vi "Minimal AR Example - Render 3D.vi"(6 "Camera Parameters":T5, 8 "error in (no error)":errorcluster, 10 "Pose":T1, 11 "ARGB Image In":T4) -> (0 "error out":errorcluster, 3 "ARGB Image Out":T4)   [LabVIEW 2020, in "examples.lvlib"]
uses:
  examples.lvlib
  common/Camera Parameters.ctl
  common/Camera Matrix.ctl
  common/Camera Distortion Coefficients.ctl
  image/ARGB Image.ctl
  ar/Pose.ctl
  ar/rvec.ctl
  ar/tvec.ctl
  image/Copy Pixmap to Image (ARGB Flatten Mask).vi
  image/Match-Value Image (Colour).vi
  image/Invert In-Place (Greyscale Bitwise).vi
  image/Copy Image (ARGB with Greyscale Mask).vi
  image/Size (ARGB).vi
  image/New Image (ARGB Preallocated).vi
  image/New Image (Greyscale Preallocated).vi
  ar/Rodrigues.vi
  ar/Rodrigues (RVec To RMat).vi
  ar/Transform Components to Transformation Matrix.vi
  <vilib>/Analysis/baseanly.llb/A x B.vi
  <vilib>/Analysis/baseanly.llb/Real A x B.vi
  image/ARGB Colour to U32 Pixel Value.vi
  image/Copy Pixmap to Image (ARGB Flatten Mask).vi/7d03ccf7-b889-4e8d-9f2a-57831e73dbde.vi
  image/Match-Value Image (Colour).vi/5701baee-35e2-4306-9a77-a9fdbb5b3a7f.vi
  image/Invert In-Place (Greyscale Bitwise).vi/821d400d-177f-4d99-a785-a8086a4d8ddd.vi
  image/Copy Image (ARGB with Greyscale Mask).vi/327a14ae-2acc-4952-87c0-fab6c3cd3da3.vi
  image/Size (ARGB).vi/69a1505b-b287-44ed-9ef9-f10ed7b260f4.vi
  image/New Image (ARGB Preallocated).vi/3321fa97-f432-4e1e-8db9-a0df79aed21b.vi
  image/New Image (Greyscale Preallocated).vi/6598b9e0-8a08-46f5-91fd-ca1b87217137.vi
  image/FixPixmap.vi
  image/Default8bitColourMap.vi
  <vilib>/Analysis/Matrix/Numeric/Conversions/Array To Matrix.vi
  <vilib>/Analysis/Matrix/Numeric/Conversions/Array To Matrix - RA2.vi
  <vilib>/Utility/error.llb/Error Cluster From Error Code.vi
  <vilib>/picture/3D Picture Control/Object/Create Object (name).vi
  <vilib>/picture/3D Picture Control/Object/Add Object (no reference).vi
  image/image.lvlib
  <vilib>/picture/3D Picture Control/NI_3D Picture Control.lvlib
  ar/ar.lvlib
  common/common.lvlib
panel:
  out "3D Canvas":refnum<vi>(3d-picture)
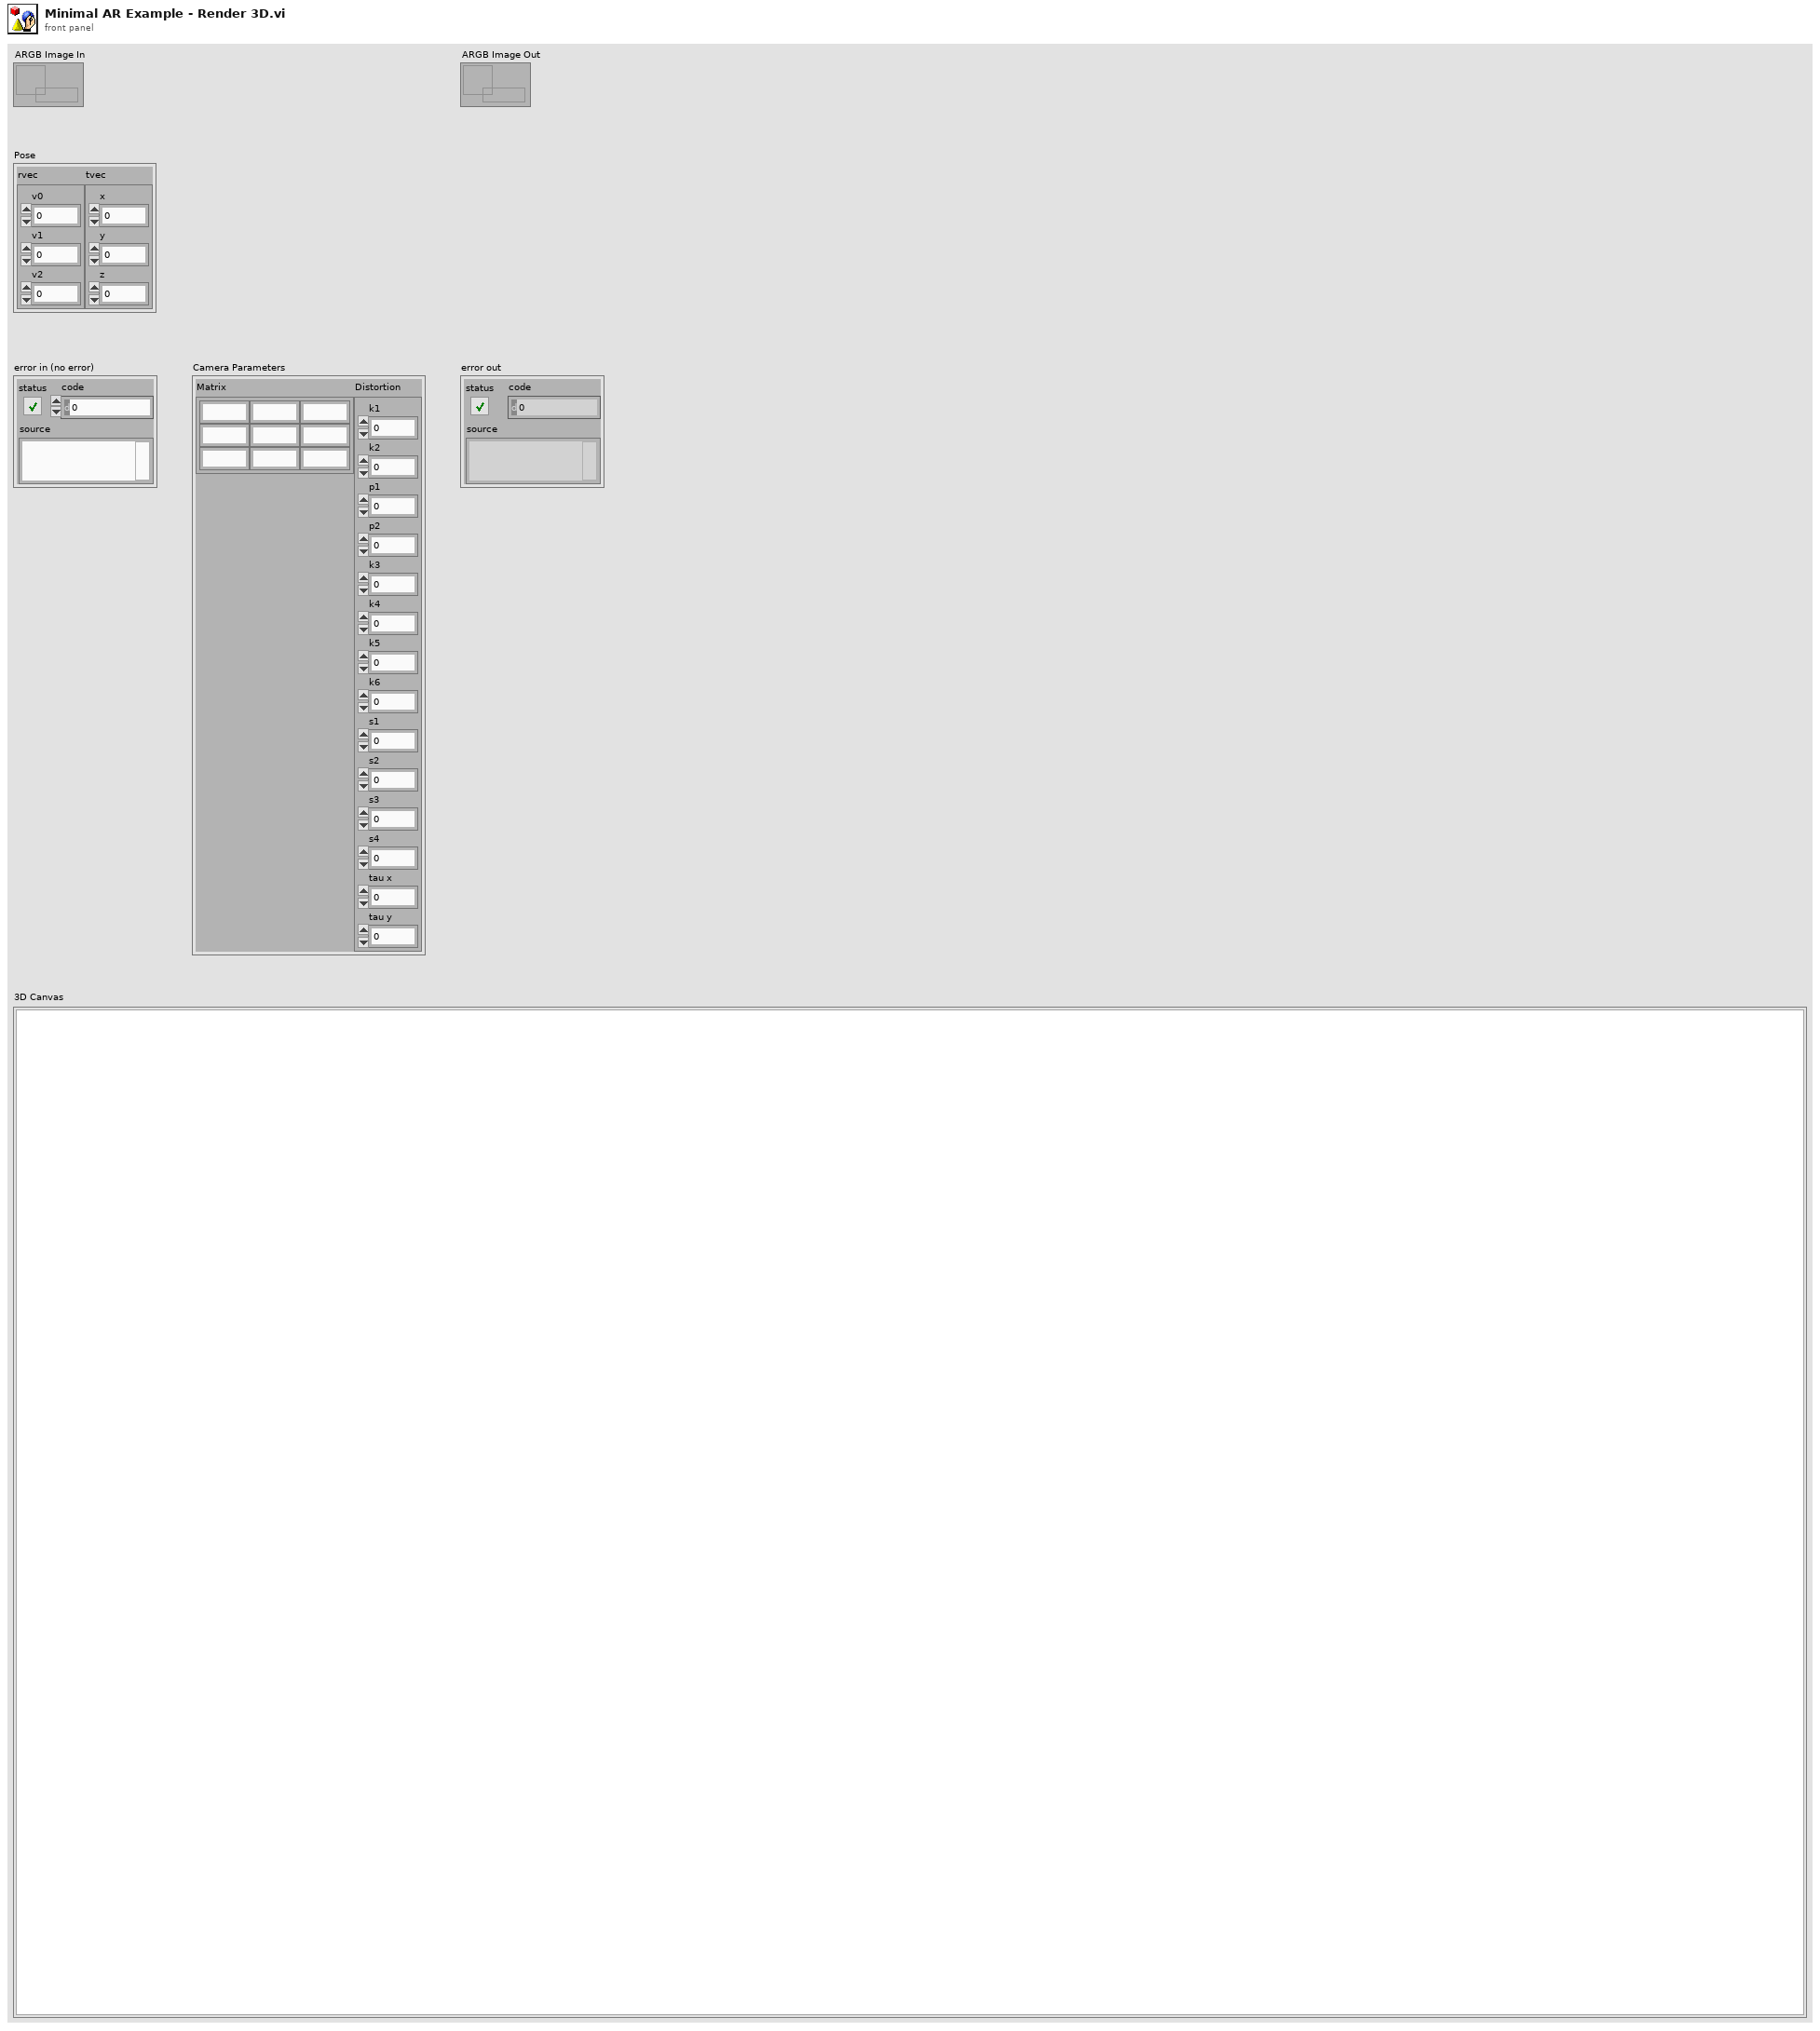
[diagram p1: front panel]
types:
  T1 = typedef "ar.lvlib/Pose.ctl" = cluster{"rvec":T2, "tvec":T3}
  T2 = typedef "ar.lvlib/rvec.ctl" = cluster{"v0":dbl, "v1":dbl, "v2":dbl}
  T3 = typedef "ar.lvlib/tvec.ctl" = cluster{"x":dbl, "y":dbl, "z":dbl}
  T4 = typedef "image.lvlib/ARGB Image.ctl" = refnum<data-value>
  T5 = typedef "common.lvlib/Camera Parameters.ctl" = cluster{"Matrix":T6, "Distortion":T7}
  T6 = typedef "common.lvlib/Camera Matrix.ctl" = cluster{"m 0,0":dbl, "m 0,1":dbl, "m 0,2":dbl, "m 1,0":dbl, "m 1,1":dbl, "m 1,2":dbl, "m 2,0":dbl, "m 2,1":dbl, "m 2,2":dbl}
  T7 = typedef "common.lvlib/Camera Distortion Coefficients.ctl" = cluster{"k1":dbl, "k2":dbl, "p1":dbl, "p2":dbl, "k3":dbl, "k4":dbl, "k5":dbl, "k6":dbl, "s1":dbl, "s2":dbl, "s3":dbl, "s4":dbl, "tau x":dbl, "tau y":dbl}
  T8 = typedef "NI_Matrix.lvlib/RealMatrix.ctl" = dbl[][]
  T9 = typedef "imagedata.ctl" = cluster{"image type":i32, "image depth":i32, "image":u8[], "mask":u8[], "colors":u32[], "Rectangle":cluster{"left":i16, "top":i16, "right":i16, "bottom":i16}}
  T10 = typedef "image.lvlib/Greyscale Image.ctl" = refnum<data-value>
  T11 = typedef "common.lvlib/Image Size (Integer).ctl" = cluster{"Width":u16, "Height":u16}
  T12 = typedef "LVBoundsTypeDef.ctl" = cluster{"Width":u32, "Height":u32}
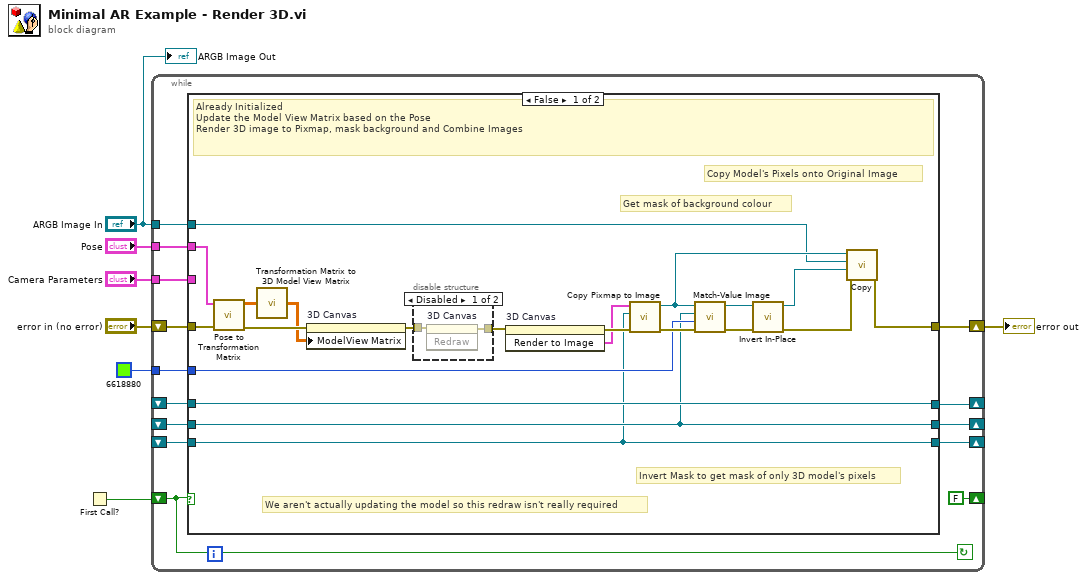
[diagram p0: block diagram]
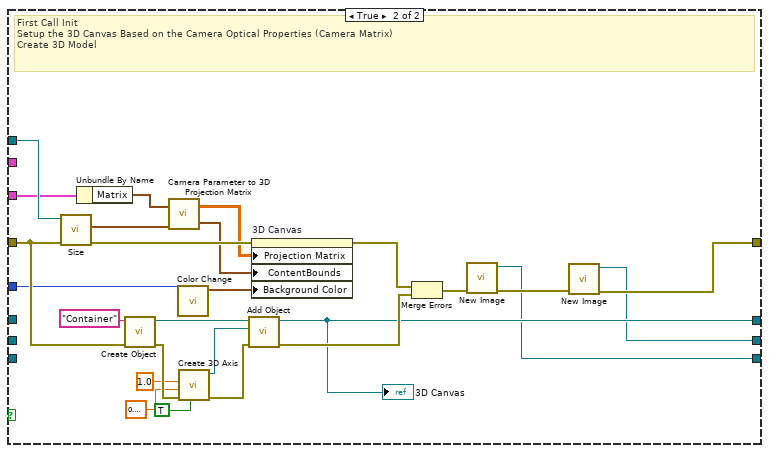
[diagram p3: hidden frame]
diagram:
  n1 = First Call?() -> (First Call?: T/F=w7:bool)
  n2 = while {
    shift-right: [FALSE ("First Call?: T/F")] -> _
    shift-left: w7 -> [w21]
    tunnel: "ARGB Image In" -> [w19]
    tunnel: "Camera Parameters" -> [w18]
    shift-right: [w14] -> w2
    shift-left: "error in (no error)" -> [w17]
    shift-right: [w16] -> _
    shift-left: _ -> [w15]
    tunnel: u32 6618880 ("Color") -> [w13]
    tunnel: "Pose" -> [w12]
    shift-right: [w11] -> _
    shift-left: _ -> [w10]
    shift-right: [w9] -> _
    shift-left: _ -> [w8]
    stop <- w21 continue-if-true
    n3 = case shown="False" w21 {
      tunnel: w19 -> [w23 w71]
      tunnel: w18 -> [_ w66]
      tunnel: w17 -> [w40 w61]
      tunnel: [w42 w54] -> w16
      tunnel: w15 -> [w42 _]
      tunnel: [w25 w51] -> w14
      tunnel: w13 -> [w31 w55]
      tunnel: w12 -> [w41 _]
      tunnel: [w27 w50] -> w11
      tunnel: w10 -> [w27 _]
      tunnel: [w28 w49] -> w9
      tunnel: w8 -> [w28 _]
      frame False {
        # "Copy Model's Pixels onto Original Image"
        # "Invert Mask to get mask of only 3D model's pixels"
        # "Get mask of background colour"
        # "We aren't actually updating the model so this redraw isn't really required"
        # "Already Initialized\nUpdate the Model View Matrix based on the Pose\nRender 3D image to Pixmap, mask background and Combine Images"
        n4 = call "Pose to Transformation Matrix.vi"("error in (no error)"=w40, "Pose"=w41) -> ("error out"=w39:errorcluster, "4x4 Transformation Matrix"=w38:T8)  [unwired: 8 in]
        n5 = call "Transformation Matrix to 3D Model View Matrix.vi"("4x4 Transformation Matrix"=w38) -> ("3D-Control Model Matrix"=w37:T8)
        n6 = property on="3D Canvas" class="SceneGraphDisp (strict)"(error in=w39, "ModelView Matrix"=w37) -> (error out=w36:errorcluster)  [unwired: 1 in, 1 out]
        n7 = disable-structure shown="Disabled" {
          disable-tunnel: w36 -> [w44 w45]
          disable-tunnel: [w43 w45] -> w35
          frame Disabled {
            n8 = invoke on="3D Canvas" class="SceneGraphDisp (strict)" method="Redraw"(error in=w44) -> (error out=w43:errorcluster)  [unwired: 2 in, 2 out]
          }
          frame Enabled {
          }
        }
        n9 = invoke on="3D Canvas" class="SceneGraphDisp (strict)" method="Render to Image"(error in=w35) -> (error out=w34:errorcluster, "Get Image"=w33:T9)  [unwired: 2 in, 1 out]
        n10 = call-poly "Copy Pixmap to Image.vi"("error in (no error)"=w34, "ARGB Image Destination in"=w27, "Pixmap Image Data"=w33) -> ("error out"=w32:errorcluster, "ARGB Image Destination"=w24:T4)  [unwired: 7 in]
        n11 = call-poly "Match-Value Image.vi"("error in (no error)"=w32, "Value"=w31, "Match in"=w28, "ARGB Image Source in"=w24) -> ("error out"=w30:errorcluster, "Match Destination"=w29:T10)  [unwired: 6 in]
        n12 = call-poly "Invert In-Place.vi"("error in (no error)"=w30, "Greyscale Image to Invert in Place in"=w29) -> ("error out"=w26:errorcluster, "Greyscale Image"=w22:T10)  [unwired: 8 in]
        n13 = call-poly "Copy.vi"("error in (no error)"=w26, "Greyscale Image Mask in"=w22, "ARGB Image Destination in"=w23, "ARGB Image Source in"=w24) -> ("error out"=w25:errorcluster)  [unwired: 6 in, 1 out]
      }
      frame True {
        # "First Call Init\nSetup the 3D Canvas Based on the Camera Optical Properties (Camera Matrix)\nCreate 3D Model"
        n14 = call-poly "Size.vi"("error in (no error)"=w61, "ARGB Image in"=w71) -> ("error out"=w64:errorcluster, "Image Size"=w67:T11)  [unwired: 7 in, 1 out]
        n15 = Unbundle By Name(w66) -> ("Matrix"=w65:T6)
        n16 = call-poly <vilib>:"Create Object.vi"("error in (no error)"=w61, "Name"="Container") -> ("error out"=w60:errorcluster, "Scene:New Object"=w69:refnum<vi>)  [unwired: 8 in]
        n17 = call "Camera Parameter to 3D Projection Matrix.vi"("Size"=w67, "Camera Matrix"=w65) -> ("Bounds"=w63:T12, "3D-Picture Projection Matrix"=w62:sgl[][])  [unwired: 2 in]
        n18 = call <vilib>:"Color Change.vi"("Color"=w55) -> ("RGBA"=w56:cluster{"R":sgl, "G":sgl, "B":sgl, "A":sgl})  [unwired: 10 in]
        n19 = call <vilib>:"Create 3D Axis.vi"("Axis label?"=TRUE, "error in (no error)"=w60, "Radius"=sgl 0.1, "Length"=sgl 1.0) -> ("error out"=w59:errorcluster, "New Object Refnum"=w68:refnum<vi>)  [unwired: 6 in]
        n20 = call-poly <vilib>:"Add Object.vi"("error in (no error)"=w59, "New Object In"=w68, "Scene Object In"=w69) -> ("error out"=w57:errorcluster, "Scene Object Out"=w54:refnum<vi>)  [unwired: 7 in]
        "3D Canvas" <- w54
        n21 = property on="3D Canvas" class="SceneGraphDisp (strict)"(error in=w64, "Projection Matrix"=w62, "ContentBounds"=w63, "Background Color"=w56) -> (error out=w58:errorcluster)  [unwired: 1 in, 1 out]
        n22 = Merge Errors(w58, w57) -> (w53:errorcluster)
        n23 = call-poly "New Image.vi"("error in (no error)"=w53) -> ("error out"=w52:errorcluster, "ARGB Image"=w50:T4)  [unwired: 9 in]
        n24 = call-poly "New Image.vi"("error in (no error)"=w52) -> ("error out"=w51:errorcluster, "Greyscale Image"=w49:T10)  [unwired: 9 in]
      }
    }
  }
  "error out" <- w2
  "ARGB Image Out" <- "ARGB Image In"
